vi "图片保存.vi"(8 "error in (no error)":errorcluster caption="错误输入（无错误）", 10 "其余文件夹名称":string[](array[string]), 11 "一维码":string) -> (0 "error out":errorcluster caption="错误输出", 2 "dup path":path caption="路径副本")   [LabVIEW 2018]
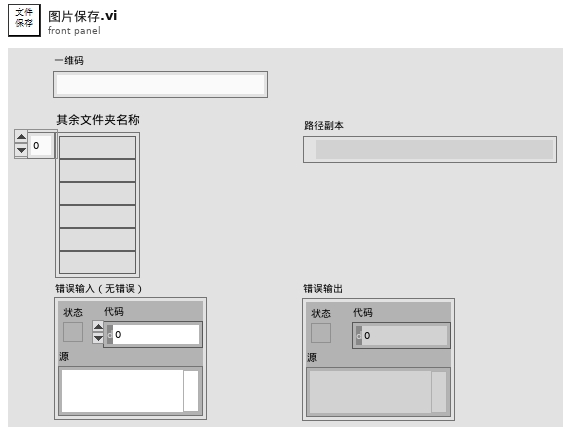
[diagram p1: front panel]
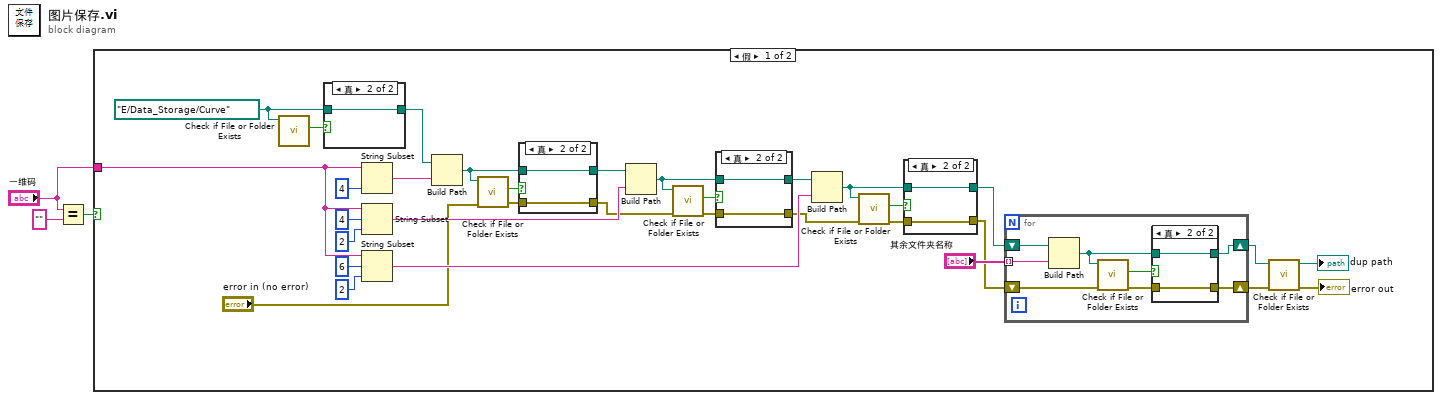
[diagram p0: block diagram]
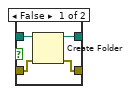
[diagram p2: hidden frame]
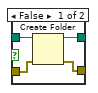
[diagram p3: hidden frame]
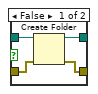
[diagram p4: hidden frame]
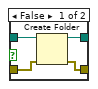
[diagram p5: hidden frame]
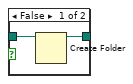
[diagram p6: hidden frame]
diagram:
  n1 = Equal?(x="一维码", y="") -> (x = y?=w2:bool)
  n2 = case shown="假" w2 {
    tunnel: "一维码" -> [w4 _]
    frame False {
      w24 = path "E:/Data_Storage/Curve" ("path")
      n3 = call <vilib>:"Check if File or Folder Exists.vi"("path"=w24) -> ("file or folder exists?"=w23:bool)  [unwired: 8 in, 2 out]
      n4 = case shown="真" w23 {
        tunnel: w24 -> [w70 w71]
        tunnel: [w69 w71] -> w25
        frame False {
          n5 = Create Folder(path (use dialog)=w70) -> (created path=w69:path)  [unwired: 2 in, 2 out]
        }
        frame True {
        }
      }
      n6 = String Subset(string=w4, length (rest)=4 ("长度（剩余）")) -> (substring=w34:string)  [unwired: 1 in]
      n7 = String Subset(string=w4, offset (0)=4 ("偏移量(0)"), length (rest)=2 ("长度（剩余）")) -> (substring=w35:string)
      n8 = String Subset(string=w4, offset (0)=6 ("偏移量(0)"), length (rest)=2 ("长度（剩余）")) -> (substring=w36:string)
      n9 = Build Path(base path=w25, name or relative path=w34) -> (appended path=w27:path)
      n10 = call <vilib>:"Check if File or Folder Exists.vi"("error in (no error)"="error in (no error)", "path"=w27) -> ("error out"=w13:errorcluster, "file or folder exists?"=w26:bool)  [unwired: 7 in, 1 out]
      n11 = case shown="真" w26 {
        tunnel: w27 -> [w66 w68]
        tunnel: [w65 w68] -> w29
        tunnel: w13 -> [w64 w67]
        tunnel: [w63 w67] -> w12
        frame False {
          n12 = Create Folder(path (use dialog)=w66, error in=w64) -> (created path=w65:path, error out=w63:errorcluster)  [unwired: 1 in, 1 out]
        }
        frame True {
        }
      }
      n13 = Build Path(base path=w29, name or relative path=w35) -> (appended path=w30:path)
      n14 = call <vilib>:"Check if File or Folder Exists.vi"("error in (no error)"=w12, "path"=w30) -> ("error out"=w11:errorcluster, "file or folder exists?"=w28:bool)  [unwired: 7 in, 1 out]
      n15 = case shown="真" w28 {
        tunnel: w30 -> [w60 w62]
        tunnel: [w59 w62] -> w33
        tunnel: w11 -> [w58 w61]
        tunnel: [w57 w61] -> w10
        frame False {
          n16 = Create Folder(path (use dialog)=w60, error in=w58) -> (created path=w59:path, error out=w57:errorcluster)  [unwired: 1 in, 1 out]
        }
        frame True {
        }
      }
      n17 = Build Path(base path=w33, name or relative path=w36) -> (appended path=w31:path)
      n18 = call <vilib>:"Check if File or Folder Exists.vi"("error in (no error)"=w10, "path"=w31) -> ("error out"=w9:errorcluster, "file or folder exists?"=w32:bool)  [unwired: 7 in, 1 out]
      n19 = case shown="真" w32 {
        tunnel: w31 -> [w54 w56]
        tunnel: [w53 w56] -> w16
        tunnel: w9 -> [w52 w55]
        tunnel: [w51 w55] -> w8
        frame False {
          n20 = Create Folder(path (use dialog)=w54, error in=w52) -> (created path=w53:path, error out=w51:errorcluster)  [unwired: 1 in, 1 out]
        }
        frame True {
        }
      }
      n21 = for {
        tunnel: "其余文件夹名称" -> [w41] mode=indexing
        shift-right: [w40] -> w5
        shift-left: w16 -> [w42]
        shift-right: [w37] -> w7
        shift-left: w8 -> [w39]
        n22 = Build Path(base path=w42, name or relative path=w41) -> (appended path=w44:path)
        n23 = call <vilib>:"Check if File or Folder Exists.vi"("error in (no error)"=w39, "path"=w44) -> ("error out"=w38:errorcluster, "file or folder exists?"=w43:bool)  [unwired: 7 in, 1 out]
        n24 = case shown="真" w43 {
          tunnel: w44 -> [w48 w50]
          tunnel: [w47 w50] -> w40
          tunnel: w38 -> [w46 w49]
          tunnel: [w45 w49] -> w37
          frame False {
            n25 = Create Folder(path (use dialog)=w48, error in=w46) -> (created path=w47:path, error out=w45:errorcluster)  [unwired: 1 in, 1 out]
          }
          frame True {
          }
        }
      }
      n26 = call <vilib>:"Check if File or Folder Exists.vi"("error in (no error)"=w7, "path"=w5) -> ("error out"=→"error out":errorcluster, "dup path"=→"dup path":path)  [unwired: 7 in, 1 out]
    }
    frame True {
    }
  }
